vi "NI VeriStand - Get Custom Device Dependencies.vi"(8 "error in (no error)":errorcluster, 11 "Device Ref in":T5 format="%.0x") -> (0 "error out":errorcluster, 2 "Dependencies":T1[](array[typedef]), 3 "Device Ref out":T5 format="%.0x")   [LabVIEW 2020, in "Custom Device API.lvlib"]
doc: "Returns all dependencies of a custom device. Dependencies are any files, such as DLLs or VIs, that the custom device requires and that you must deploy to the target along with the custom device."
uses:
  <vilib>/NI VeriStand/Custom Device API/Custom Device API.lvlib
  <vilib>/NI VeriStand/Custom Device API/Custom Device Item Ref.ctl
  <vilib>/NI VeriStand/Custom Device API/Custom Device File Dependency.ctl
  <vilib>/NI VeriStand/Custom Device API/Path Specification.ctl
  <vilib>/NI VeriStand/Custom Device API/Path Type.ctl
  <vilib>/NI VeriStand/Custom Device API/Custom Device Supported Target.ctl
  e3914414-f99c-44de-8638-3ead00e755da.vi
  <vilib>/NI VeriStand/Custom Device API/Custom Device Offline Path.vi
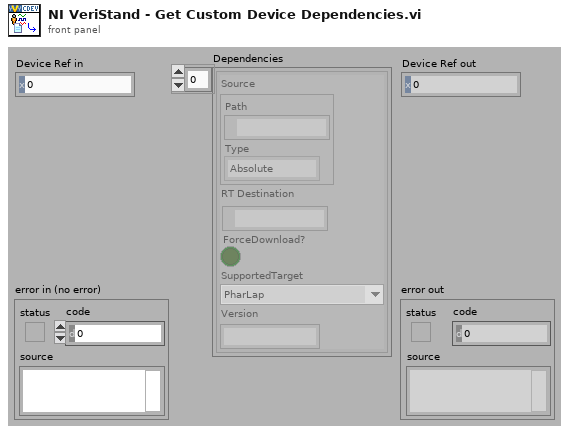
[diagram p1: front panel]
types:
  T1 = typedef "Custom Device API.lvlib/Custom Device File Dependency.ctl" = cluster{"Source":T2, "RT Destination":path, "ForceDownload?":bool, "SupportedTarget":T4, "Version":string}
  T2 = typedef "Custom Device API.lvlib/Path Specification.ctl" = cluster{"Path":path, "Type":T3}
  T3 = typedef "Custom Device API.lvlib/Path Type.ctl" = enum16{"Absolute", "To Base", "To Common Data Dir", "To Application Data Dir"}
  T4 = typedef "Custom Device API.lvlib/Custom Device Supported Target.ctl" = enum16{"All", "PharLap", "VxWorks", "Windows", "Linux_32_ARM", "Linux_x64", "PharLap & Windows", "PharLap & VxWorks", "VxWorks & Windows"}
  T5 = typedef "Custom Device API.lvlib/Custom Device Item Ref.ctl" = u64
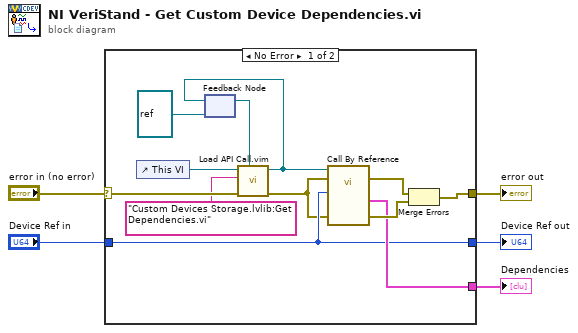
[diagram p0: block diagram]
diagram:
  n1 = case shown="No Error" "error in (no error)" {
    selector: "error in (no error)" -> [w10 w19]
    tunnel: [w16 w19] -> w5
    tunnel: [w14 w18] -> w4
    tunnel: "Device Ref in" -> [w14 w18]
    tunnel: [w15 _] -> w2
    frame No Error {
      n2 = control-ref of="This VI"() -> (w12:refnum<vi>)
      n3 = feedback #1(refnum<vi> refnum ("type specifier VI Refnum (for type only)")) -> (w13:refnum<vi>)
      n4 = call "Load API Call.vim"("VI reference in"=w13, "error in (no error)"=w10, "VI qualified name"="Custom Devices Storage.lvlib:Get Dependencies.vi", "Caller VI ref"=w12) -> ("error out"=w9:errorcluster, "VI reference"=w11:refnum<vi>)  [unwired: 6 in]
      n5 = feedback-in #1(w11) -> ()
      n6 = call-by-ref "?"(reference=w11, error in=w9, 8:"error in (no error)"=w9, "Device Ref in"=w14) -> (error out=w6:errorcluster, 0:"error out"=w17:errorcluster, "Dependencies"=w15:T1[])  [unwired: 7 in, 2 out]
      n7 = Merge Errors(w6, w17) -> (w16:errorcluster)
    }
    frame Error {
    }
  }
  "Device Ref out" <- w4
  "error out" <- w5
  "Dependencies" <- w2
